vi "Read from TXT.vi"(17 "Файл с параметрами":path) -> (0 "Кол-во циклов наслаивания":dbl, 1 "Кол-во используемых растворов":dbl, 2 "Кол-во погружений в каждый раствор:":dbl[](array[numeric]), 3 "Опускания подложки в растворе:":dbl[](array[numeric]), 4 "Глубина погружения в раствор [мм]:":dbl[](array[numeric]), 5 "Опускания подложки до раствора:":dbl[](array[numeric]), 6 "Режим погружения":i32=33, 7 "Высота подложки [мм]":dbl, 8 "Подъем подложки над раствором:":dbl[](array[numeric]), 9 "Кол-во жидкости в стакане [мл]:":dbl[](array[numeric]), 10 "Подъема подложки из раствора:":dbl[](array[numeric]), 12 "Нахождения в растворе:":dbl[](array[numeric]), 14 "Высота стакана [мм]":dbl, 15 "Задержки после подъема из раствора:":dbl[](array[numeric]), 16 "Температура в стаканах:":dbl[](array[numeric]), 19 "Время всего процесса":timestamp=timestamp(-10799.315441346698 s since 1904-01-01) format="%<%H:%M:%S>T")   [LabVIEW 2016]
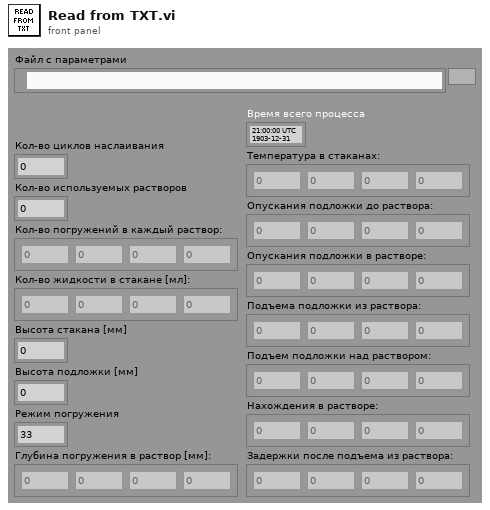
[diagram p1: front panel]
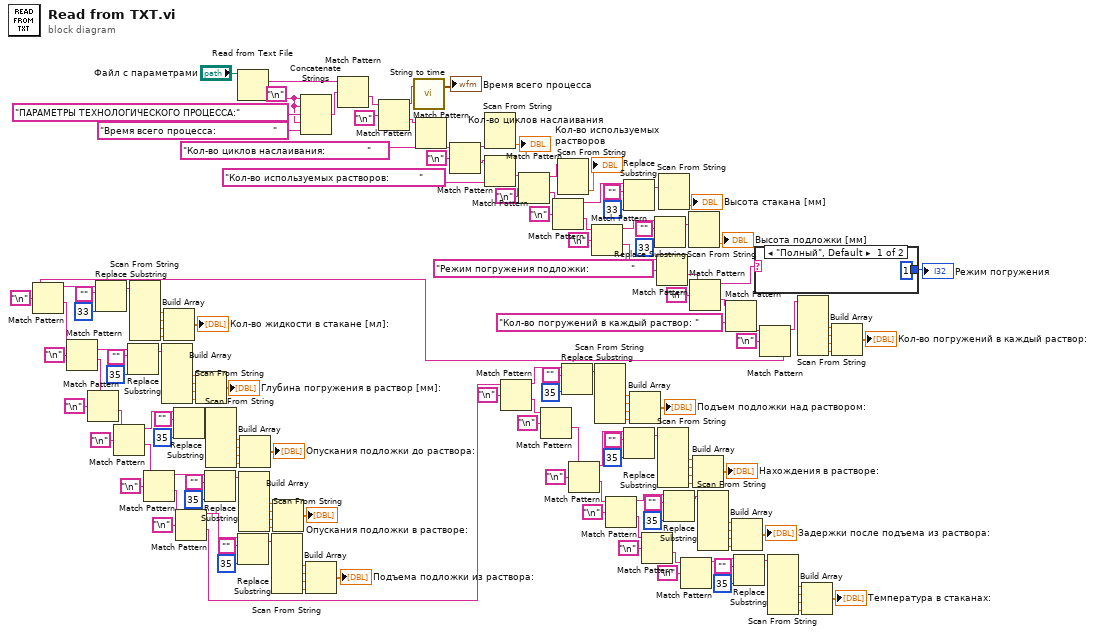
[diagram p0: block diagram]
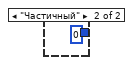
[diagram p2: hidden frame]
diagram:
  w153 = "\n"
  n1 = Read from Text File(file (use dialog)="Файл с параметрами") -> (text=w156:string)  [unwired: 3 in, 3 out]
  n2 = Concatenate Strings(w153, w153, "ПАРАМЕТРЫ ТЕХНОЛОГИЧЕСКОГО ПРОЦЕССА:" ("string"), w153, "Время всего процесса:                   " ("string")) -> (w155:string)
  n3 = Match Pattern(string=w156, regular expression=w155) -> (after substring=w151:string)  [unwired: 1 in, 3 out]
  n4 = Match Pattern(string=w151, regular expression="\n") -> (before substring=w149:string, after substring=w147:string)  [unwired: 1 in, 2 out]
  n5 = call "String to time.vi"("Строка со временем"=w149) -> ("Время всего процесса"=→"Время всего процесса":timestamp)  [unwired: 1 in, 1 out]
  n6 = Match Pattern(string=w147, regular expression="Кол-во циклов наслаивания:              " ("string")) -> (after substring=w144:string)  [unwired: 1 in, 3 out]
  n7 = Match Pattern(string=w144, regular expression="\n") -> (before substring=w143:string, after substring=w139:string)  [unwired: 1 in, 2 out]
  n8 = Scan From String(input string=w143) -> (output 1=→"Кол-во циклов наслаивания":dbl)  [unwired: 4 in, 3 out]
  n9 = Match Pattern(string=w139, regular expression="Кол-во используемых растворов:          " ("string")) -> (after substring=w140:string)  [unwired: 1 in, 3 out]
  n10 = Match Pattern(string=w140, regular expression="\n") -> (before substring=w136:string, after substring=w129:string)  [unwired: 1 in, 2 out]
  n11 = Match Pattern(string=w129, regular expression="\n") -> (before substring=w133:string, after substring=w122:string)  [unwired: 1 in, 2 out]
  n12 = Scan From String(input string=w136) -> (output 1=→"Кол-во используемых растворов":dbl)  [unwired: 4 in, 3 out]
  n13 = Match Pattern(string=w122, regular expression="\n") -> (before substring=w126:string, after substring=w121:string)  [unwired: 1 in, 2 out]
  n14 = Replace Substring(2:33 ("length (len. of substring)"), 4:"", 5:w133) -> (1:w132:string)  [unwired: 1 in, 1 out]
  n15 = Replace Substring(2:33 ("length (len. of substring)"), 4:"", 5:w126) -> (1:w125:string)  [unwired: 1 in, 1 out]
  n16 = Match Pattern(string=w121, regular expression="Режим погружения подложки:              " ("string")) -> (after substring=w118:string)  [unwired: 1 in, 3 out]
  n17 = Scan From String(input string=w132) -> (output 1=→"Высота стакана [мм]":dbl)  [unwired: 4 in, 3 out]
  n18 = Scan From String(input string=w125) -> (output 1=→"Высота подложки [мм]":dbl)  [unwired: 4 in, 3 out]
  n19 = Match Pattern(string=w118, regular expression="\n") -> (before substring=w117:string, after substring=w115:string)  [unwired: 1 in, 2 out]
  n20 = Match Pattern(string=w115, regular expression="Кол-во погружений в каждый раствор: " ("string")) -> (after substring=w112:string)  [unwired: 1 in, 3 out]
  n21 = case shown="\"Полный\", Default" w117 {
    tunnel: [1 0] -> w116
    frame "Полный", Default {
    }
    frame "Частичный" {
    }
  }
  "Режим погружения" <- w116
  n22 = Match Pattern(string=w112, regular expression="\n") -> (before substring=w111:string, after substring=w102:string)  [unwired: 1 in, 2 out]
  n23 = Match Pattern(string=w102, regular expression="\n") -> (before substring=w101:string, after substring=w93:string)  [unwired: 1 in, 2 out]
  n24 = Match Pattern(string=w93, regular expression="\n") -> (before substring=w4:string, after substring=w91:string)  [unwired: 1 in, 2 out]
  n25 = Match Pattern(string=w91, regular expression="\n") -> (after substring=w82:string)  [unwired: 1 in, 3 out]
  n26 = Replace Substring(2:33 ("length (len. of substring)"), 4:"", 5:w101) -> (1:w95:string)  [unwired: 1 in, 1 out]
  n27 = Match Pattern(string=w82, regular expression="\n") -> (before substring=w81:string, after substring=w69:string)  [unwired: 1 in, 2 out]
  n28 = Replace Substring(2:35 ("length (len. of substring)"), 4:"", 5:w4) -> (1:w5:string)  [unwired: 1 in, 1 out]
  n29 = Scan From String(input string=w95) -> (output 1=w100:dbl, output 2=w99:dbl, output 3=w98:dbl, output 4=w97:dbl)  [unwired: 7 in, 3 out]
  n30 = Match Pattern(string=w69, regular expression="\n") -> (before substring=w71:string, after substring=w58:string)  [unwired: 1 in, 2 out]
  n31 = Scan From String(input string=w5) -> (output 1=w7:dbl, output 2=w6:dbl, output 3=w2:dbl, output 4=w1:dbl)  [unwired: 7 in, 3 out]
  n32 = Build Array(w100, w99, w98, w97) -> (→"Кол-во жидкости в стакане [мл]:":dbl[])
  n33 = Replace Substring(2:35 ("length (len. of substring)"), 4:"", 5:w81) -> (1:w84:string)  [unwired: 1 in, 1 out]
  n34 = Match Pattern(string=w58, regular expression="\n") -> (before substring=w60:string, after substring=w48:string)  [unwired: 1 in, 2 out]
  n35 = Build Array(w7, w6, w2, w1) -> (→"Глубина погружения в раствор [мм]:":dbl[])
  n36 = Replace Substring(2:35 ("length (len. of substring)"), 4:"", 5:w71) -> (1:w73:string)  [unwired: 1 in, 1 out]
  n37 = Scan From String(input string=w84) -> (output 1=w88:dbl, output 2=w87:dbl, output 3=w86:dbl, output 4=w80:dbl)  [unwired: 7 in, 3 out]
  n38 = Replace Substring(2:35 ("length (len. of substring)"), 4:"", 5:w60) -> (1:w62:string)  [unwired: 1 in, 1 out]
  n39 = Scan From String(input string=w73) -> (output 1=w77:dbl, output 2=w76:dbl, output 3=w75:dbl, output 4=w70:dbl)  [unwired: 7 in, 3 out]
  n40 = Build Array(w88, w87, w86, w80) -> (→"Опускания подложки до раствора:":dbl[])
  n41 = Scan From String(input string=w62) -> (output 1=w66:dbl, output 2=w65:dbl, output 3=w64:dbl, output 4=w59:dbl)  [unwired: 7 in, 3 out]
  n42 = Build Array(w77, w76, w75, w70) -> (→"Опускания подложки в растворе:":dbl[])
  n43 = Build Array(w66, w65, w64, w59) -> (→"Подъема подложки из раствора:":dbl[])
  n44 = Match Pattern(string=w48, regular expression="\n") -> (before substring=w50:string, after substring=w35:string)  [unwired: 1 in, 2 out]
  n45 = Match Pattern(string=w35, regular expression="\n") -> (after substring=w34:string)  [unwired: 1 in, 3 out]
  n46 = Replace Substring(2:35 ("length (len. of substring)"), 4:"", 5:w50) -> (1:w47:string)  [unwired: 1 in, 1 out]
  n47 = Match Pattern(string=w34, regular expression="\n") -> (before substring=w39:string, after substring=w23:string)  [unwired: 1 in, 2 out]
  n48 = Scan From String(input string=w47) -> (output 1=w55:dbl, output 2=w54:dbl, output 3=w53:dbl, output 4=w49:dbl)  [unwired: 7 in, 3 out]
  n49 = Match Pattern(string=w23, regular expression="\n") -> (before substring=w26:string, after substring=w21:string)  [unwired: 1 in, 2 out]
  n50 = Replace Substring(2:35 ("length (len. of substring)"), 4:"", 5:w39) -> (1:w37:string)  [unwired: 1 in, 1 out]
  n51 = Build Array(w55, w54, w53, w49) -> (→"Подъем подложки над раствором:":dbl[])
  n52 = Match Pattern(string=w21, regular expression="\n") -> (after substring=w10:string)  [unwired: 1 in, 3 out]
  n53 = Scan From String(input string=w37) -> (output 1=w44:dbl, output 2=w43:dbl, output 3=w42:dbl, output 4=w38:dbl)  [unwired: 7 in, 3 out]
  n54 = Replace Substring(2:35 ("length (len. of substring)"), 4:"", 5:w26) -> (1:w24:string)  [unwired: 1 in, 1 out]
  n55 = Match Pattern(string=w10, regular expression="\n") -> (before substring=w13:string)  [unwired: 1 in, 3 out]
  n56 = Build Array(w44, w43, w42, w38) -> (→"Нахождения в растворе:":dbl[])
  n57 = Scan From String(input string=w24) -> (output 1=w31:dbl, output 2=w30:dbl, output 3=w29:dbl, output 4=w25:dbl)  [unwired: 7 in, 3 out]
  n58 = Build Array(w31, w30, w29, w25) -> (→"Задержки после подъема из раствора:":dbl[])
  n59 = Replace Substring(2:35 ("length (len. of substring)"), 4:"", 5:w13) -> (1:w11:string)  [unwired: 1 in, 1 out]
  n60 = Scan From String(input string=w11) -> (output 1=w18:dbl, output 2=w17:dbl, output 3=w16:dbl, output 4=w12:dbl)  [unwired: 7 in, 3 out]
  n61 = Scan From String(input string=w111) -> (output 1=w110:dbl, output 2=w109:dbl, output 3=w108:dbl, output 4=w107:dbl)  [unwired: 7 in, 3 out]
  n62 = Build Array(w18, w17, w16, w12) -> (→"Температура в стаканах:":dbl[])
  n63 = Build Array(w110, w109, w108, w107) -> (→"Кол-во погружений в каждый раствор:":dbl[])
